vi "DB Variant To Data_XSFP_86To85.vi"(10 "Version-State Cluster In":T1, 11 "XRef":refnum<vi>) -> (0 "Custom Label":string, 1 "Custom Warning To Issue":string, 2 "Version-State Cluster Out":T1, 3 "Action":T2)   [LabVIEW 2013]
uses:
  <vilib>/XSFPSupport/SFPChangeStateAction.ctl
  <vilib>/XSFPSupport/NI_XSFPSupport.lvlib
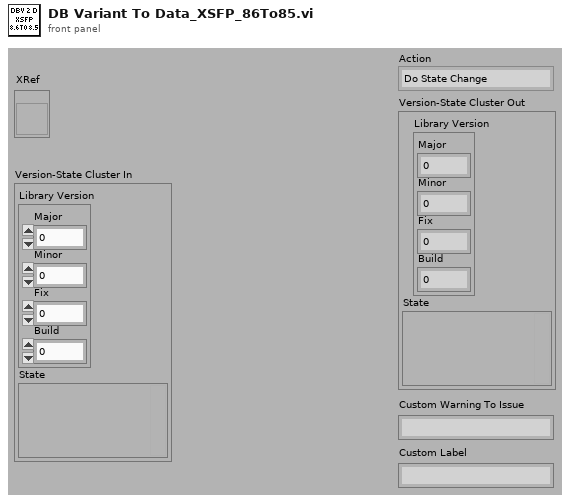
[diagram p1: front panel]
types:
  T1 = cluster{"Library Version":cluster{"Major":u16, "Minor":u16, "Fix":u16, "Build":u16}, "State":variant}
  T2 = typedef "NI_XSFPSupport.lvlib/SFPChangeStateAction.ctl" = enum32{"Do State Change", "Replace With Label", "Fail SFP"}
  T3 = cluster{"Major":u16, "Minor":u16, "Fix":u16, "Build":u16}
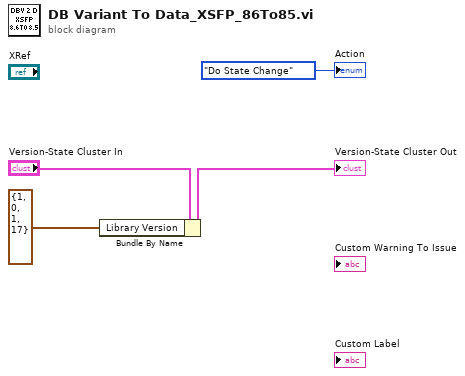
[diagram p0: block diagram]
diagram:
  n1 = Bundle By Name(cluster="Version-State Cluster In", "Library Version"=T3 {"Major"=1, "Minor"=0, "Fix"=1, "Build"=17}) -> (→"Version-State Cluster Out":T1)
  "Action" <- SFPChangeStateAction."Do State Change" ("Action")
